vi "HDM3065B.vi"(4 "error in":T14, 7 "Command":T15) -> (0 "error out":T14, 3 "Response":T12)   [LabVIEW 2018]
uses:
  MOKO_LabViewLibrary/MokoLowLevel/MokoLowLovelControl/MLLC_Command.ctl
  MOKO_LabViewLibrary/MokoLowLevel/MokoLowLovelControl/MLLC_Error.ctl
  MOKO_LabViewLibrary/MokoLowLevel/MokoLowLovelControl/MLLC_Mode.ctl
  MOKO_LabViewLibrary/MokoLowLevel/MokoLowLovelControl/MLLC_Response.ctl
  MOKO_LabViewLibrary/MokoLowLevel/MokoLowLovelControl/MLLC_DriverName.ctl
  MOKO_LabViewLibrary/MokoLowLevel/MokoLowLovelControl/MLLC_Request.ctl
  MOKO_LabViewLibrary/MokoLowLevel/MokoLowLovelControl/MLLC_ErrorCode.ctl
  MOKO_LabViewLibrary/MokoLowLevel/MokoLowLovelControl/MLLC_ResponseInit.ctl
  MOKO_LabViewLibrary/MokoLowLevel/MokoLowLovelControl/MLLC_ConnectCluster.ctl
  MOKO_LabViewLibrary/MokoLowLevel/MokoLowLovelControl/MLLC_InterfaceType.ctl
  MOKO_LabViewLibrary/MokoLowLevel/MokoLowLovelControl/MLLC_OpenedSession.ctl
  MOKO_LabViewLibrary/MokoLowLevel/MokoLowLovelControl/MLLC_InterfaceSettings.ctl
  MOKO_LabViewLibrary/MokoLowLevel/MokoLowLovelControl/MLLC_InterfaceKind.ctl
  data/HDM3065B_Functions.ctl
panel:
  in  "Settings":T8={"Saved Data"=variant, "Data"={"Connect"={"InterfaceType"=enum."VISA", "OpenedSession"="", "InterfaceSettings"={"Interface"=enum."GPIB", "EOS 4 read"=enum."LF (\\n)", "EOS 4 write"=enum."LF (\\n)", "TMO, ms"=5000, "Sett"=variant(cluster{"Baud Rate":u32, "Data Bits":u16, "Parity":u16, "Stop Bits":u16, "Flow Control":u16, "Eho":bool} {"Baud Rate"=75, "Data Bits"=0, "Parity"=0, "Stop Bits"=0, "Flow Control"=0, "Eho"=FALSE})}}, "Channel"=1, "Func"=enum."VDC"}}
  in  "Response Init array":T9="HEWLETT-PACKARD,34401A,0,9-4-1"
  in  "Error Code":T6=5475
  in  "Request":T10="*idn?"
  in  "Driver Name":T11="HDM3065B_GERMAN"
  in  "Mode":T13=enum."Check"
  # "SCPI = MEASure:VOLTage:DC?"
  # "SCPI = SENSe:VOLTage :RANGe 20"
  # "SCPI = SENSe:VOLTage :RANGe MAX"
  # "SCPI = MEASure:VOLTage:DC?"
  # "SCPI = VOLTage :RANGe MAX"
  # "HDM3065B CUSTOM DRIVER GERMAN"
  # "MEASure | FETCh2\n:ENABle <n>\n:ARRay :CURRent?1\n:NTRansition <n>\n :VOLTage?1"
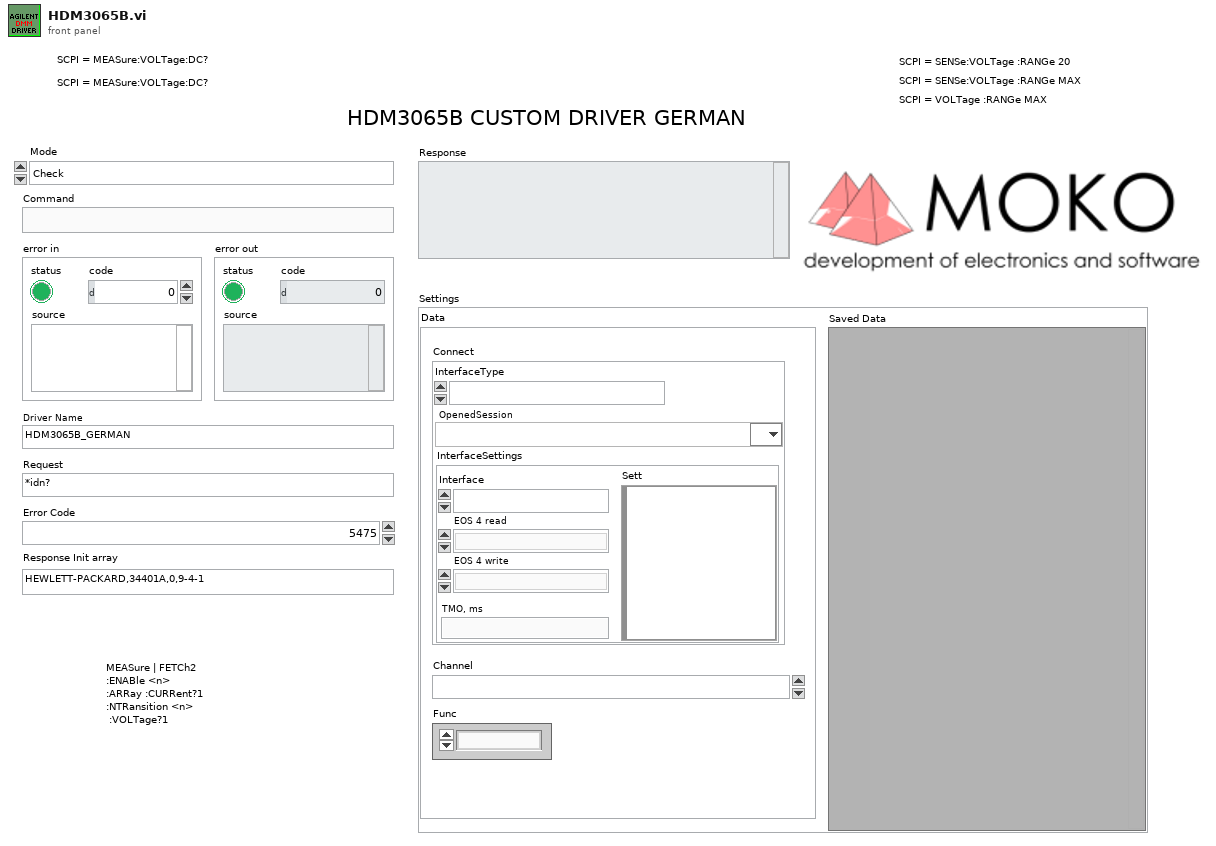
[diagram p1: front panel]
types:
  T1 = typedef "MLLC_ConnectCluster.ctl" = cluster{"InterfaceType":T2, "OpenedSession":T3, "InterfaceSettings":T4}
  T2 = typedef "MLLC_InterfaceType.ctl" = enum16{"VISA", "Prologix USB-GPIB"}
  T3 = typedef "MLLC_OpenedSession.ctl" = refnum<visa-resource-name>
  T4 = typedef "MLLC_InterfaceSettings.ctl" = cluster{"Interface":T5, "EOS 4 read":enum16{"Default (=EOS 4 write)", "CR (\\r)", "LF (\\n)", "None"}, "EOS 4 write":enum16{"CR+LF (\\r\\n)", "CR (\\r)", "LF (\\n)", "None"}, "TMO, ms":i32, "Sett":variant}
  T5 = typedef "MLLC_InterfaceKind.ctl" = enum16{"RS232", "GPIB", "USB", "Ethernet", "another"}
  T6 = typedef "MLLC_ErrorCode.ctl" = u32
  T7 = typedef "HDM3065B_Functions.ctl" = enum16{"VDC", "VAC", "IDC", "IAC", "F", "R2", "R4", "CAP"}
  T8 = cluster{"Saved Data":variant, "Data":cluster{"Connect":T1, "Channel":T6, "Func":T7}}
  T9 = typedef "MLLC_ResponseInit.ctl" = string
  T10 = typedef "MLLC_Request.ctl" = string
  T11 = typedef "MLLC_DriverName.ctl" = string
  T12 = typedef "MLLC_Response.ctl" = string
  T13 = typedef "MLLC_Mode.ctl" = enum16{"get", "set", "close", "Init", "Check"}
  T14 = typedef "MLLC_Error.ctl" = errorcluster
  T15 = typedef "MLLC_Command.ctl" = string
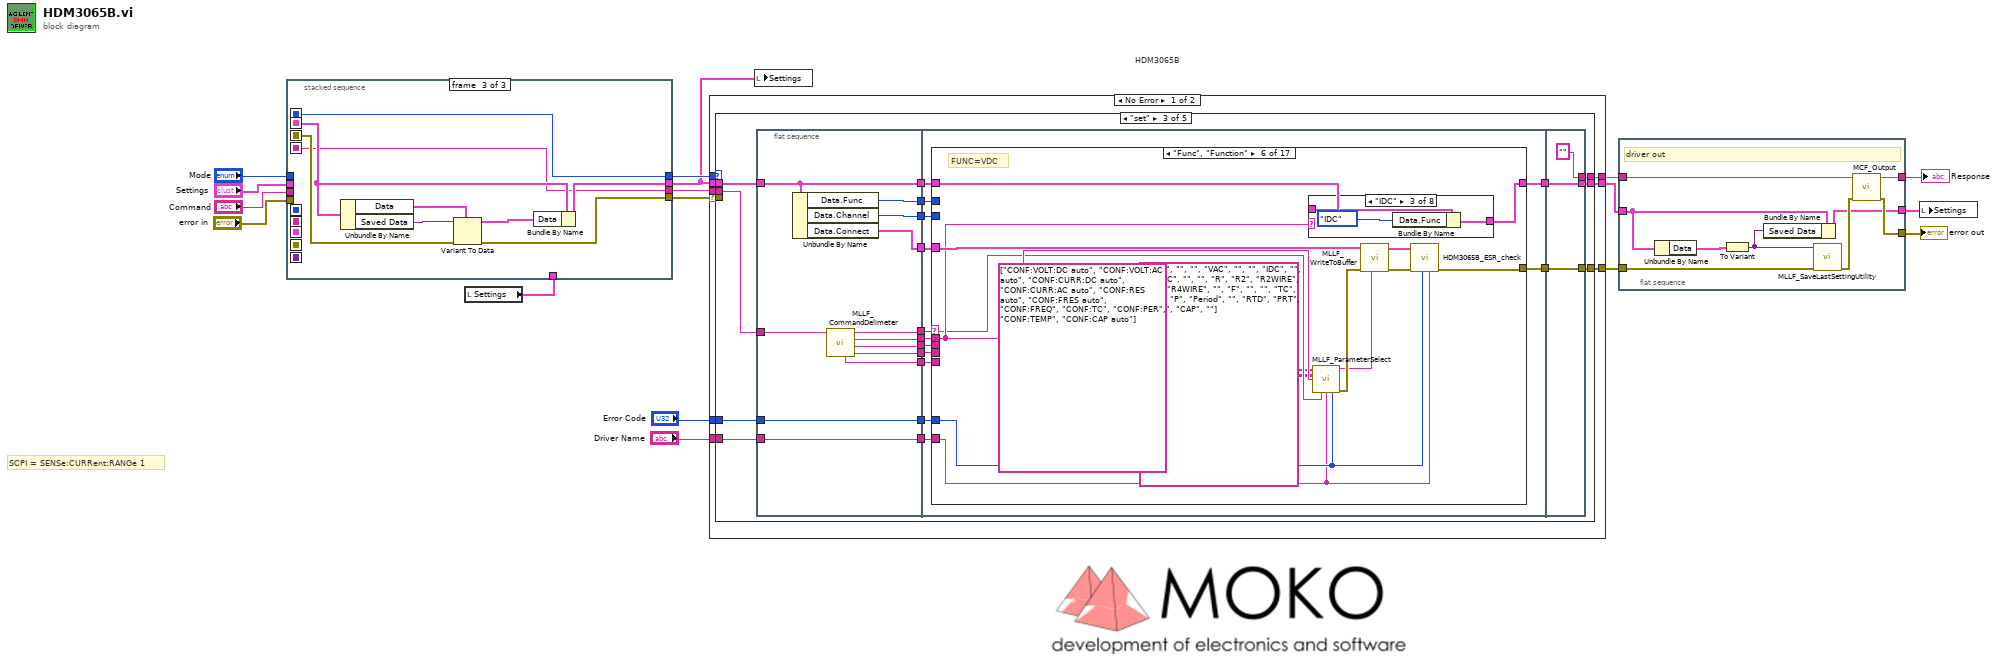
[diagram p0: block diagram]
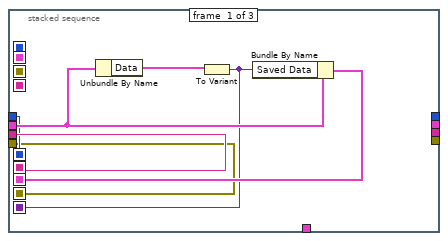
[diagram p2: hidden frame]
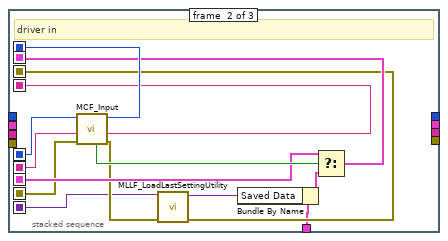
[diagram p3: hidden frame]
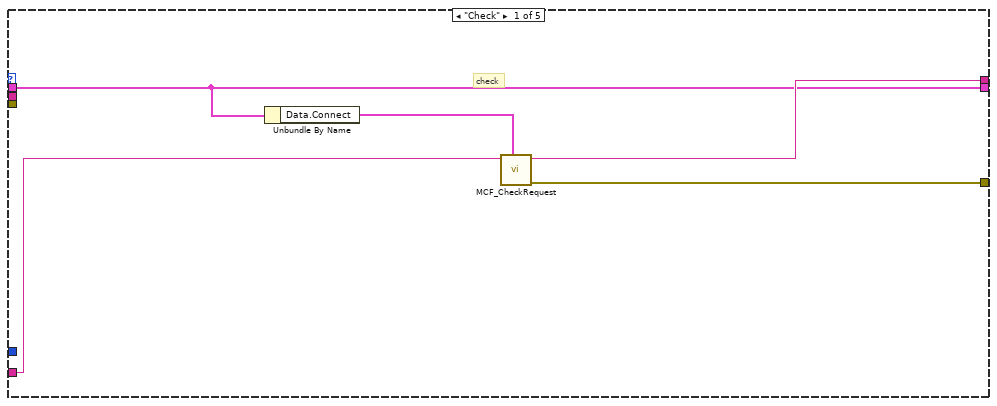
[diagram p4: hidden frame]
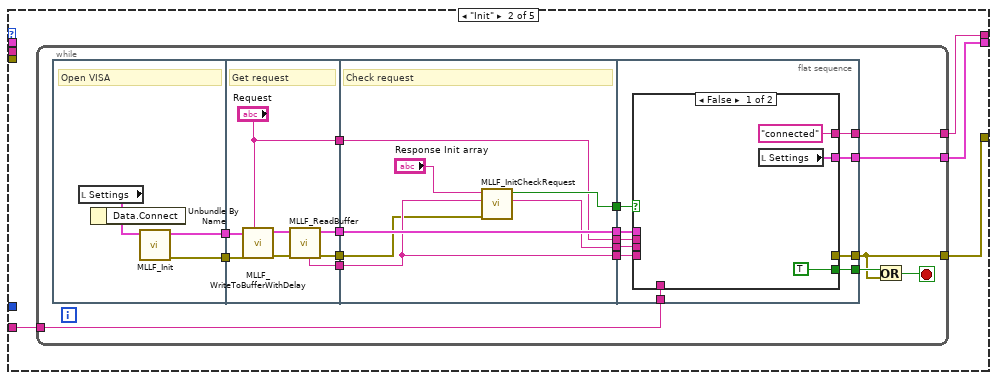
[diagram p5: hidden frame]
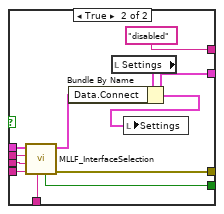
[diagram p6: hidden frame]
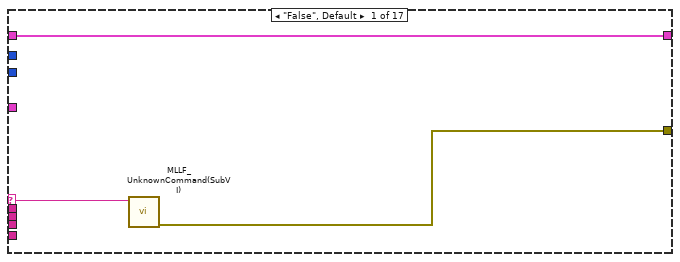
[diagram p7: hidden frame]
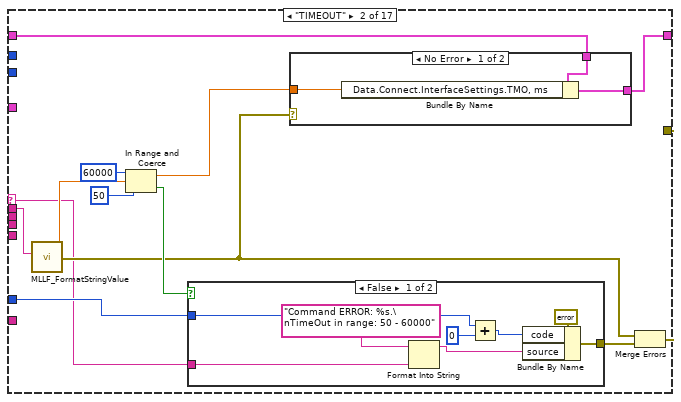
[diagram p8: hidden frame]
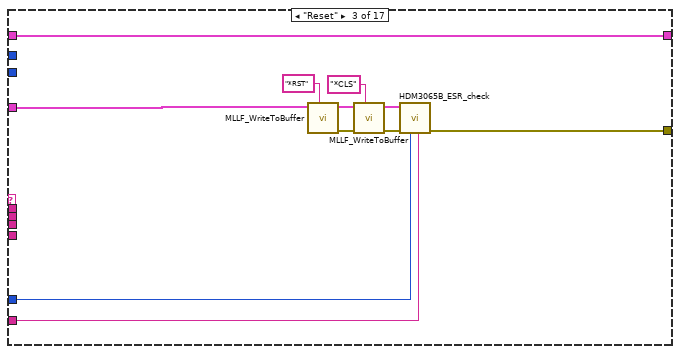
[diagram p11: hidden frame]
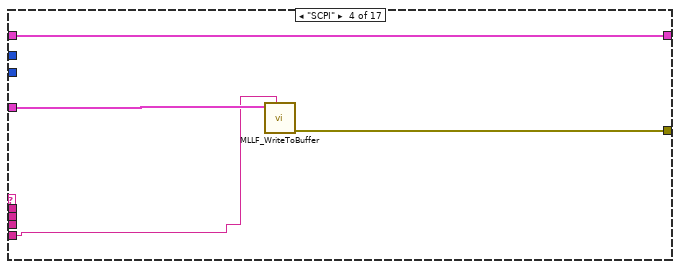
[diagram p12: hidden frame]
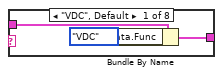
[diagram p14: hidden frame]
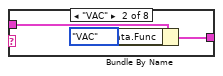
[diagram p15: hidden frame]
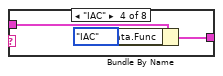
[diagram p16: hidden frame]
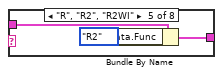
[diagram p17: hidden frame]
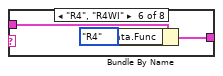
[diagram p18: hidden frame]
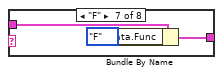
[diagram p19: hidden frame]
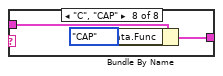
[diagram p20: hidden frame]
diagram:
  # "SCPI = SENSe:CURRent:RANGe 1"
  # "HDM3065B"
  n1 = local read "Settings"() -> (w8:T8)
  n2 = stacked-sequence {
    seq-local: [w20 _ _] -> [_ w36 _]
    seq-local: [w19 _ _] -> [_ w37 _]
    seq-local: [w22 _ _] -> [_ w32 _]
    seq-local: [w18 _ _] -> [_ w31 _]
    seq-local: [w21 _ _] -> [_ w27 _]
    seq-local: [_ w28 _] -> [_ _ w44]
    seq-local: [_ w38 _] -> [_ _ w41]
    seq-local: [_ w35 _] -> [_ _ w40]
    seq-local: [_ w34 _] -> [_ _ w45]
    tunnel: "Command" -> [w20 _ _]
    tunnel: "Mode" -> [w19 _ _]
    tunnel: "error in" -> [w18 _ _]
    tunnel: "Settings" -> [w23 _ _]
    tunnel: w8 -> [_ w26 _]
    tunnel: [_ _ w40] -> w10
    tunnel: [_ _ w43] -> w1
    tunnel: [_ _ w42] -> w9
    tunnel: [_ _ w41] -> w11
    frame #0 {
      n3 = Unbundle By Name(w23) -> ("Data"=w24:cluster{"Connect":T1, "Channel":T6, "Func":T7})
      n4 = To Variant(anything=w24) -> (Variant=w21:variant)
      n5 = Bundle By Name(cluster=w23, "Saved Data"=w21) -> (w22:T8)
    }
    frame #1 {
      # "driver in"
      n6 = call "MCF_Input.vi"("Error In"=w31, "Command in"=w36, "Mode in"=w37) -> ("Error Out"=w30:errorcluster, "Command out"=w35:string, "Mode out"=w38:T13, "Boolean"=w33:bool)  [unwired: 5 in]
      n7 = call "MLLF_LoadLastSettingUtility.vi"("Error In"=w30, "Save data in"=w27) -> ("Error Out"=w28:errorcluster, "Save data out"=w25:variant)  [unwired: 8 in]
      n8 = Bundle By Name(cluster=w26, "Saved Data"=w25) -> (w29:T8)
      n9 = Select(t=w32, s=w33, f=w29) -> (s? t:f=w34:T8)
    }
    frame #2 {
      n10 = Unbundle By Name(w45) -> ("Data"=w46:cluster{"Connect":T1, "Channel":T6, "Func":T7}, "Saved Data"=w39:variant)
      n11 = Variant To Data(error in=w44, type=w46, Variant=w39) -> (data=w47:cluster{"Connect":T1, "Channel":T6, "Func":T7}, error out=w42:errorcluster)
      n12 = Bundle By Name(cluster=w45, "Data"=w47) -> (w43:T8)
    }
  }
  n13 = case shown="No Error" w9 {
    selector: w9 -> [w53 w607]
    tunnel: [w54 w607] -> w5
    tunnel: w11 -> [w56 _]
    tunnel: [w55 "An error occurred in the driver input module." ("String")] -> w7
    tunnel: w10 -> [w48 _]
    tunnel: w1 -> [w49 w606]
    tunnel: "Error Code" -> [w52 _]
    tunnel: "Driver Name" -> [w51 _]
    tunnel: [w50 w606] -> w6
    frame No Error {
      n14 = case shown="\"set\"" w56 {
        tunnel: [w60 w65 w139 w529 "" ("String")] -> w55
        tunnel: [w61 w63 w142 w530 w603] -> w54
        tunnel: w53 -> [_ _ _ w544 _]
        tunnel: w52 -> [_ _ w145 w546 _]
        tunnel: w51 -> [w59 w62 w143 w545 _]
        tunnel: [w57 w64 w144 w547 w602] -> w50
        tunnel: w49 -> [w57 _ w128 w535 w602]
        tunnel: w48 -> [_ _ w127 w534 _]
        frame "Check" {
          # "check"
          n15 = Unbundle By Name(w57) -> ("Data.Connect"=w58:T1)
          n16 = call "MCF_CheckRequest.vi"("Permanent data.Connect"=w58, "Driver Name"=w59) -> ("Error Out"=w61:errorcluster, "Output String"=w60:string)  [unwired: 8 in]
        }
        frame "Init" {
          n17 = while {
            tunnel: [w71] -> w63
            tunnel: [w70] -> w65
            tunnel: [w69] -> w64
            tunnel: w62 -> [w73]
            stop <- w82 stop-if-true
            n18 = flat-sequence {
              tunnel: [w86] -> w81
              tunnel: [w85] -> w80
              tunnel: w81 -> [w92]
              tunnel: w80 -> [w91]
              tunnel: [w90] -> w79
              tunnel: [w89] -> w78
              tunnel: [w88] -> w77
              tunnel: ["Request"] -> w67
              tunnel: w79 -> [w98]
              tunnel: w78 -> [w101]
              tunnel: w77 -> [w100]
              tunnel: [w101] -> w76
              tunnel: [w100] -> w75
              tunnel: [w97] -> w74
              tunnel: [w96] -> w68
              tunnel: w67 -> [w95]
              tunnel: [w95] -> w66
              tunnel: w76 -> [w110]
              tunnel: w75 -> [w109]
              tunnel: w74 -> [w111]
              tunnel: w73 -> [w108]
              tunnel: [w107] -> w72
              tunnel: [w106] -> w71
              tunnel: [w105] -> w70
              tunnel: [w104] -> w69
              tunnel: w68 -> [w103]
              tunnel: w66 -> [w102]
              frame #0 {
                # "Open VISA"
                n19 = local read "Settings"() -> (w84:T8)
                n20 = Unbundle By Name(w84) -> ("Data.Connect"=w83:T1)
                n21 = call "MLLF_Init.vi"("DriverConnect in"=w83) -> ("Error Out"=w86:errorcluster, "DriverConnect out"=w85:T1)  [unwired: 7 in]
              }
              frame #1 {
                # "Get request"
                n22 = call "MLLF_WriteToBufferWithDelay.vi"("Command"="Request", "Error In"=w92, "DriverConnect in"=w91) -> ("Error Out"=w93:errorcluster, "DriverConnect out"=w94:T1)  [unwired: 7 in]
                n23 = call "MLLF_ReadBuffer.vi"("Error In"=w93, "DriverConnect in"=w94) -> ("Error Out"=w90:errorcluster, "DriverConnect out"=w89:T1, "String"=w88:string)  [unwired: 6 in]
              }
              frame #2 {
                # "Check request"
                n24 = call "MLLF_InitCheckRequest.vi"("error in (no error)"=w98, "Answer"=w100, "Response Init"="Response Init array") -> ("ResponseInit out"=w96:string, "Design"=w97:bool)  [unwired: 5 in, 2 out]
              }
              frame #3 {
                n25 = case shown="False" w111 {
                  tunnel: w110 -> [_ w124]
                  tunnel: [TRUE w119] -> w107
                  tunnel: [_ w122] -> w106
                  tunnel: ["connected" "disabled"] -> w105
                  tunnel: [w112 w120] -> w104
                  tunnel: w109 -> [_ w117]
                  tunnel: w108 -> [_ w118]
                  tunnel: w103 -> [_ w116]
                  tunnel: w102 -> [_ w115]
                  frame False {
                    n26 = local read "Settings"() -> (w112:T8)
                  }
                  frame True {
                    n27 = call "MLLF_InterfaceSelection.vi"("Driver Name"=w118, "Answer:"=w117, "Response"=w116, "Request"=w115, "DriverConnect in"=w124) -> ("error out"=w122:T14, "DriverConnect out"=w123:T1, "stop init?"=w119:bool)  [unwired: 2 in, 2 out]
                    n28 = local read "Settings"() -> (w125:T8)
                    n29 = Bundle By Name(cluster=w125, "Data.Connect"=w123) -> (w120:T8)
                    n30 = local write "Settings"(w120) -> ()
                  }
                }
              }
            }
            n31 = Or(x=w72, y=w71) -> (x .or. y?=w82:bool)
          }
        }
        frame "set" {
          n32 = flat-sequence {
            tunnel: w143 -> [w156]
            tunnel: w128 -> [w147]
            tunnel: w145 -> [w157]
            tunnel: [w157] -> w138
            tunnel: [w147] -> w137
            tunnel: [w156] -> w136
            tunnel: [w153] -> w135
            tunnel: [w154] -> w134
            tunnel: [w155] -> w133
            tunnel: [w148] -> w132
            tunnel: [w149] -> w131
            tunnel: [w150] -> w130
            tunnel: [w151] -> w129
            tunnel: w127 -> [w152]
            tunnel: [w146] -> w126
            tunnel: [w168] -> w141
            tunnel: [w161] -> w140
            tunnel: w138 -> [w170]
            tunnel: w137 -> [w169]
            tunnel: w136 -> [w167]
            tunnel: w135 -> [w166]
            tunnel: w134 -> [w165]
            tunnel: w133 -> [w164]
            tunnel: w132 -> [w163]
            tunnel: w131 -> [w162]
            tunnel: w130 -> [w160]
            tunnel: w129 -> [w159]
            tunnel: w126 -> [w158]
            tunnel: [w527] -> w142
            tunnel: [w528] -> w144
            tunnel: w141 -> [w528]
            tunnel: w140 -> [w527]
            tunnel: ["" ("String")] -> w139
            frame #0 {
              n33 = Unbundle By Name(w147) -> ("Data.Func"=w155:T7, "Data.Channel"=w154:T6, "Data.Connect"=w153:T1)
              n34 = call "MLLF_CommandDelimeter.vi"("command with param"=w152) -> ("param 3"=w151:string, "param 2"=w150:string, "param 1"=w149:string, "command"=w148:string, "Spit delimetre"=w146:string)  [unwired: 6 in]
            }
            frame #1 {
              n35 = case shown="\"Func\", \"Function\"" w163 {
                selector: w163 -> [w172 w175 _ _ _ w221 _ _ _ _ _ _ w441 w448 w474 w500 w513]
                tunnel: w162 -> [_ w174 _ _ _ w222 w270 _ w303 w318 w365 w399 w442 w449 w475 w501 w514]
                tunnel: [w171 w180 w200 w210 _ w226 w253 _ w307 w336 w369 w403 w446 w470 w496 w509 w520] -> w161
                tunnel: w170 -> [_ w181 w202 _ _ w228 _ _ w306 w335 w368 w402 w443 w453 w479 w505 w522]
                tunnel: w169 -> [w173 w185 w209 w213 w214 w224 w272 w284 w308 w337 w370 w404 w447 w471 w497 w510 w525]
                tunnel: [w173 w186 w209 w213 w214 w223 w272 w284 w308 w337 w370 w404 w447 w471 w497 w510 w525] -> w168
                tunnel: w166 -> [_ _ w199 w212 _ w225 w271 _ w304 w333 w366 w400 w445 w469 w495 w503 w518]
                tunnel: w167 -> [_ _ w201 _ _ w227 _ _ w305 w334 w367 w401 w444 w454 w480 w506 w521]
                tunnel: w165 -> [_ _ _ _ _ _ _ _ _ _ _ _ _ _ _ _ _]
                tunnel: w164 -> [_ _ _ _ _ _ _ _ _ _ _ _ _ _ _ _ _]
                tunnel: w160 -> [_ _ _ _ _ _ _ _ _ _ _ _ _ _ _ _ _]
                tunnel: w159 -> [_ _ _ _ _ _ _ _ _ _ _ _ _ _ _ _ _]
                tunnel: w158 -> [_ _ _ w211 _ _ _ _ _ _ _ _ _ _ _ _ _]
                frame "False", Default {
                  n36 = call "MLLF_UnknownCommand(SubVI).vi"("Unknown command"=w172) -> ("error out"=w171:errorcluster)  [unwired: 10 in]
                }
                frame "TIMEOUT" {
                  n37 = call "MLLF_FormatStringValue.vi"("String Value"=w174) -> ("error out"=w176:T14, "number"=w177:dbl)  [unwired: 8 in, 1 out]
                  n38 = In Range and Coerce(upper limit=60000, x=w177, lower limit=50) -> (coerced(x)=w182:dbl, In Range?=w178:bool)
                  n39 = case shown="False" w178 {
                    tunnel: [w193 _] -> w179
                    tunnel: w181 -> [w192 _]
                    tunnel: w175 -> [w191 _]
                    frame False {
                      n40 = Format Into String(format string="Command ERROR: %s.\nTimeOut in range: 50 - 60000", w191) -> (resulting string=w195:string)  [unwired: 2 in, 1 out]
                      n41 = Add(x=w192, y=0) -> (x+y=w196:T6)
                      n42 = Bundle By Name(cluster=errorcluster {"status"=TRUE, "code"=0, "source"=""} ("error out"), "code"=w196, "source"=w195) -> (w193:errorcluster)
                    }
                    frame True {
                    }
                  }
                  n43 = case shown="No Error" w176 {
                    tunnel: [w189 w190] -> w186
                    tunnel: w185 -> [w188 w190]
                    tunnel: w182 -> [w187 _]
                    frame No Error {
                      n44 = Bundle By Name(cluster=w188, "Data.Connect.InterfaceSettings.TMO, ms"=w187) -> (w189:T8)
                    }
                    frame Error {
                    }
                  }
                  n45 = Merge Errors(w176, w179) -> (w180:errorcluster)
                }
                frame "Reset" {
                  n46 = call "MLLF_WriteToBuffer.vi"("String"="*RST", "DriverConnect in"=w199) -> ("error out"=w207:T14, "DriverConnect out"=w208:T1)  [unwired: 6 in]
                  n47 = call "MLLF_WriteToBuffer.vi"("String"="*CLS" ("write buffer"), "error in"=w207, "DriverConnect in"=w208) -> ("error out"=w204:T14, "DriverConnect out"=w203:T1)  [unwired: 5 in]
                  n48 = call "HDM3065B_ESR_check.vi"("Driver Name"=w201, "Error Code"=w202, "error in"=w204, "DriverConnect in"=w203) -> ("error out"=w200:T14)  [unwired: 6 in, 1 out]
                }
                frame "SCPI" {
                  n49 = call "MLLF_WriteToBuffer.vi"("String"=w211, "DriverConnect in"=w212) -> ("error out"=w210:T14)  [unwired: 6 in, 1 out]
                }
                frame "<----MAIN FUNCTIONS---->" {
                }
                frame "Func", "Function" {
                  # "FUNC=VDC"
                  n50 = case shown="\"IDC\"" w222 {
                    tunnel: w224 -> [w231 w234 w237 w240 w243 w246 w249 w252]
                    tunnel: [w230 w233 w236 w239 w242 w245 w248 w251] -> w223
                    frame "VDC", Default {
                      n51 = Bundle By Name(cluster=w231, "Data.Func"=HDM3065B_Functions."VDC" ("Func")) -> (w230:T8)
                    }
                    frame "VAC" {
                      n52 = Bundle By Name(cluster=w234, "Data.Func"=HDM3065B_Functions."VAC" ("Func")) -> (w233:T8)
                    }
                    frame "IDC" {
                      n53 = Bundle By Name(cluster=w237, "Data.Func"=HDM3065B_Functions."IDC" ("Func")) -> (w236:T8)
                    }
                    frame "IAC" {
                      n54 = Bundle By Name(cluster=w240, "Data.Func"=HDM3065B_Functions."IAC" ("Func")) -> (w239:T8)
                    }
                    frame "R", "R2", "R2WI" {
                      n55 = Bundle By Name(cluster=w243, "Data.Func"=HDM3065B_Functions."R2" ("Func")) -> (w242:T8)
                    }
                    frame "R4", "R4WI" {
                      n56 = Bundle By Name(cluster=w246, "Data.Func"=HDM3065B_Functions."R4" ("Func")) -> (w245:T8)
                    }
                    frame "F" {
                      n57 = Bundle By Name(cluster=w249, "Data.Func"=HDM3065B_Functions."F" ("Func")) -> (w248:T8)
                    }
                    frame "C", "CAP" {
                      n58 = Bundle By Name(cluster=w252, "Data.Func"=HDM3065B_Functions."CAP" ("Func")) -> (w251:T8)
                    }
                  }
                  n59 = call "MLLF_ParameterSelect.vi"("Command to equipment"=string[] ["CONF:VOLT:DC auto", "CONF:VOLT:AC auto", "CONF:CURR:DC auto", "CONF:CURR:AC auto", "CONF:RES auto", "CONF:FRES auto", "CONF:FREQ", "CONF:TC", "CONF:PER", "CONF:TEMP", "CONF:CAP auto"] ("Names"), "Names"=string[][] [["VDC", "", ""], ["VAC", "", ""], ["IDC", "", ""], ["IAC", "", ""], ["R", "R2", "R2WIRE"], ["R4", "R4WIRE", ""], ["F", "", ""], ["TC", "", ""], ["P", "Period", ""], ["RTD", "PRT", ""], ["C", "CAP", ""]], "Input"=w222, "Command"=w221, "Driver Name"=w227, "Error Code"=w228) -> ("Choice"=w215:string, "Error Out"=w216:errorcluster)  [unwired: 8 in]
                  n60 = call "MLLF_WriteToBuffer.vi"("String"=w215, "error in"=w216, "DriverConnect in"=w225) -> ("error out"=w220:T14, "DriverConnect out"=w219:T1)  [unwired: 5 in]
                  n61 = call "HDM3065B_ESR_check.vi"("Driver Name"=w227, "Error Code"=w228, "error in"=w220, "DriverConnect in"=w219) -> ("error out"=w226:T14)  [unwired: 6 in, 1 out]
                }
                frame "Range" {
                  w258 = TRUE ("replace all? (F)")
                  n62 = call "MLLF_WriteToBuffer.vi"("String"="CONFigure? ", "DriverConnect in"=w271) -> ("error out"=w266:T14, "DriverConnect out"=w267:T1)  [unwired: 6 in]
                  n63 = call "MLLF_ReadBuffer.vi"("Error In"=w266, "DriverConnect in"=w267) -> ("Error Out"=w255:errorcluster, "DriverConnect out"=w265:T1, "String"=w260:string)  [unwired: 6 in]
                  n64 = case shown="\"False\", Default" w270 {
                    selector: w270 -> [w274 _ _ _]
                    tunnel: [w277 w278 w280 w282] -> w269
                    tunnel: [w276 "RANG:AUTO ON" ("String") "RANG MIN" ("String") "RANG MAX" ("String")] -> w263
                    tunnel: w255 -> [w273 w278 w280 w282]
                    frame "False", Default {
                      n65 = call "MLLF_FormatStringValue.vi"("error in"=w273, "String Value"=w274, "Format"="RANG %#e" ("format string")) -> ("error out"=w277:T14, "String Value Formated"=w276:T15)  [unwired: 6 in, 1 out]
                    }
                    frame "Auto" {
                    }
                    frame "MIN" {
                    }
                    frame "MAX" {
                    }
                  }
                  n66 = Search and Replace String(replace all?=w258, case sensitive?=w258, input string=w260, search string="\"") -> (result string=w259:string)  [unwired: 4 in, 3 out]
                  n67 = Match Pattern(string=w259, regular expression="[\\s\\t]+") -> (before substring=w261:string)  [unwired: 1 in, 3 out]
                  n68 = Concatenate Strings("SENSe:" ("string"), w261, ":" ("string"), w263) -> (w256:string)
                  n69 = call "MLLF_WriteToBuffer.vi"("String"=w256, "error in"=w269, "DriverConnect in"=w265) -> ("error out"=w253:T14)  [unwired: 5 in, 1 out]
                }
                frame "---------ADDITIONAL---------" {
                }
                frame "Res", "Resolution" {
                  w288 = TRUE ("replace all? (F)")
                  n70 = call "MLLF_WriteToBuffer.vi"("String"="CONFigure? ", "DriverConnect in"=w304) -> ("error out"=w297:T14, "DriverConnect out"=w298:T1)  [unwired: 6 in]
                  n71 = call "MLLF_ReadBuffer.vi"("Error In"=w297, "DriverConnect in"=w298) -> ("Error Out"=w296:errorcluster, "DriverConnect out"=w295:T1, "String"=w290:string)  [unwired: 6 in]
                  n72 = Search and Replace String(replace all?=w288, case sensitive?=w288, input string=w290, search string="\"") -> (result string=w289:string)  [unwired: 4 in, 3 out]
                  n73 = case shown="\"MIN\"" w303 {
                    selector: w303 -> [w310 _ _]
                    tunnel: [w313 w314 w316] -> w302
                    tunnel: [w312 "RES MAX" ("String") "RES MIN" ("String")] -> w293
                    tunnel: w296 -> [w309 w314 w316]
                    frame "False", Default {
                      n74 = call "MLLF_FormatStringValue.vi"("error in"=w309, "String Value"=w310, "Format"="RES %#e" ("format string")) -> ("error out"=w313:T14, "String Value Formated"=w312:T15)  [unwired: 6 in, 1 out]
                    }
                    frame "MAX" {
                    }
                    frame "MIN" {
                    }
                  }
                  n75 = Match Pattern(string=w289, regular expression="[\\s\\t]+") -> (before substring=w291:string)  [unwired: 1 in, 3 out]
                  n76 = Concatenate Strings("SENSe:" ("string"), w291, ":" ("string"), w293) -> (w286:string)
                  n77 = call "MLLF_WriteToBuffer.vi"("String"=w286, "error in"=w302, "DriverConnect in"=w295) -> ("error out"=w301:T14, "DriverConnect out"=w300:T1)  [unwired: 5 in]
                  n78 = call "HDM3065B_ESR_check.vi"("Driver Name"=w305, "Error Code"=w306, "error in"=w301, "DriverConnect in"=w300) -> ("error out"=w307:T14)  [unwired: 6 in, 1 out]
                }
                frame "Aper", "Aperture", "MeasTime" {
                  w321 = TRUE ("replace all? (F)")
                  n79 = call "MLLF_WriteToBuffer.vi"("String"="CONFigure? ", "DriverConnect in"=w333) -> ("error out"=w330:T14, "DriverConnect out"=w331:T1)  [unwired: 6 in]
                  n80 = call "MLLF_ReadBuffer.vi"("Error In"=w330, "DriverConnect in"=w331) -> ("Error Out"=w329:errorcluster, "DriverConnect out"=w328:T1, "String"=w323:string)  [unwired: 6 in]
                  n81 = Search and Replace String(replace all?=w321, case sensitive?=w321, input string=w323, search string="\"") -> (result string=w322:string)  [unwired: 4 in, 3 out]
                  n82 = case shown="\"OFF\"" w318 {
                    selector: w318 -> [w342 _]
                    tunnel: [w345 w346] -> w340
                    tunnel: [w344 "APER:ENAB OFF" ("String")] -> w326
                    tunnel: w329 -> [w341 w346]
                    frame "False", Default {
                      n83 = call "MLLF_FormatStringValue.vi"("error in"=w341, "String Value"=w342, "Format"="APER %#e" ("format string")) -> ("error out"=w345:T14, "String Value Formated"=w344:T15)  [unwired: 6 in, 1 out]
                    }
                    frame "OFF" {
                    }
                  }
                  n84 = Match Pattern(string=w322, regular expression="[\\s\\t]+") -> (before substring=w324:string)  [unwired: 1 in, 3 out]
                  n85 = Concatenate Strings(w324, ":" ("string"), w326) -> (w319:string)
                  n86 = call "MLLF_WriteToBuffer.vi"("String"=w319, "error in"=w340, "DriverConnect in"=w328) -> ("error out"=w339:T14, "DriverConnect out"=w338:T1)  [unwired: 5 in]
                  n87 = call "HDM3065B_ESR_check.vi"("Driver Name"=w334, "Error Code"=w335, "error in"=w339, "DriverConnect in"=w338) -> ("error out"=w336:T14)  [unwired: 6 in, 1 out]
                }
                frame "IntegrationTime", "IntTime", "NPLC" {
                  w351 = TRUE ("replace all? (F)")
                  n88 = call "MLLF_WriteToBuffer.vi"("String"="CONFigure? ", "DriverConnect in"=w366) -> ("error out"=w359:T14, "DriverConnect out"=w360:T1)  [unwired: 6 in]
                  n89 = call "MLLF_ReadBuffer.vi"("Error In"=w359, "DriverConnect in"=w360) -> ("DriverConnect out"=w358:T1, "String"=w353:string)  [unwired: 6 in, 1 out]
                  n90 = Search and Replace String(replace all?=w351, case sensitive?=w351, input string=w353, search string="\"") -> (result string=w352:string)  [unwired: 4 in, 3 out]
                  n91 = case shown="Default" w365 {
                    tunnel: [w374 w378 w382] -> w364
                    tunnel: [w373 w377 w381] -> w356
                    tunnel: w365 -> [w371 w375 w379]
                    frame Default {
                      n92 = call "MLLF_FormatStringValue.vi"("String Value"=w371, "Format"="NPLC %#e" ("format string")) -> ("error out"=w374:T14, "String Value Formated"=w373:T15)  [unwired: 7 in, 1 out]
                    }
                    frame "MIN" {
                      n93 = call "MLLF_FormatStringValue.vi"("String Value"=w375, "Format"="NPLC MIN" ("format string")) -> ("error out"=w378:T14, "String Value Formated"=w377:T15)  [unwired: 7 in, 1 out]
                    }
                    frame "MAX" {
                      n94 = call "MLLF_FormatStringValue.vi"("String Value"=w379, "Format"="NPLC MAX" ("format string")) -> ("error out"=w382:T14, "String Value Formated"=w381:T15)  [unwired: 7 in, 1 out]
                    }
                  }
                  n95 = Match Pattern(string=w352, regular expression="[\\s\\t]+") -> (before substring=w354:string)  [unwired: 1 in, 3 out]
                  n96 = Concatenate Strings("SENSe:" ("string"), w354, ":" ("string"), w356) -> (w349:string)
                  n97 = call "MLLF_WriteToBuffer.vi"("String"=w349, "error in"=w364, "DriverConnect in"=w358) -> ("error out"=w363:T14, "DriverConnect out"=w362:T1)  [unwired: 5 in]
                  n98 = call "HDM3065B_ESR_check.vi"("Driver Name"=w367, "Error Code"=w368, "error in"=w363, "DriverConnect in"=w362) -> ("error out"=w369:T14)  [unwired: 6 in, 1 out]
                }
                frame "ACBand", "ACBandwidth", "Band", "Bandwidth" {
                  w386 = TRUE ("replace all? (F)")
                  n99 = call "MLLF_WriteToBuffer.vi"("String"="CONFigure? ", "DriverConnect in"=w400) -> ("error out"=w393:T14, "DriverConnect out"=w394:T1)  [unwired: 6 in]
                  n100 = call "MLLF_ReadBuffer.vi"("Error In"=w393, "DriverConnect in"=w394) -> ("Error Out"=w392:errorcluster, "DriverConnect out"=w391:T1, "String"=w388:string)  [unwired: 6 in]
                  n101 = case shown="\"MAX\"" w399 {
                    tunnel: [w409 w414 w419] -> w398
                    tunnel: w392 -> [w408 w413 w418]
                    tunnel: [w407 w412 w417] -> w389
                    tunnel: w399 -> [w405 w410 w415]
                    frame Default {
                      n102 = call "MLLF_FormatStringValue.vi"("error in"=w408, "String Value"=w405, "Format"="BAND %#f" ("format string")) -> ("error out"=w409:T14, "String Value Formated"=w407:T15)  [unwired: 6 in, 1 out]
                    }
                    frame "MAX" {
                      n103 = call "MLLF_FormatStringValue.vi"("error in"=w413, "String Value"=w410, "Format"="BAND MAX" ("format string")) -> ("error out"=w414:T14, "String Value Formated"=w412:T15)  [unwired: 6 in, 1 out]
                    }
                    frame "MIN" {
                      n104 = call "MLLF_FormatStringValue.vi"("error in"=w418, "String Value"=w415, "Format"="BAND MIN" ("format string")) -> ("error out"=w419:T14, "String Value Formated"=w417:T15)  [unwired: 6 in, 1 out]
                    }
                  }
                  n105 = Search and Replace String(replace all?=w386, case sensitive?=w386, input string=w388, search string="\"") -> (result string=w387:string)  [unwired: 4 in, 3 out]
                  n106 = Match Pattern(string=w387, regular expression="[\\s\\t]+") -> ()  [unwired: 1 in, 4 out]
                  n107 = Concatenate Strings(":DET:" ("string"), w389) -> (w384:string)
                  n108 = call "MLLF_WriteToBuffer.vi"("String"=w384, "error in"=w398, "DriverConnect in"=w391) -> ("error out"=w397:T14, "DriverConnect out"=w396:T1)  [unwired: 5 in]
                  n109 = call "HDM3065B_ESR_check.vi"("Driver Name"=w401, "Error Code"=w402, "error in"=w397, "DriverConnect in"=w396) -> ("error out"=w403:T14)  [unwired: 6 in, 1 out]
                }
                frame "AutoZero", "ZERO" {
                  w429 = TRUE ("replace all? (F)")
                  n110 = call "MLLF_WriteToBuffer.vi"("String"="CONFigure? ", "DriverConnect in"=w445) -> ("error out"=w436:T14, "DriverConnect out"=w437:T1)  [unwired: 6 in]
                  n111 = call "MLLF_ReadBuffer.vi"("Error In"=w436, "DriverConnect in"=w437) -> ("Error Out"=w423:errorcluster, "DriverConnect out"=w435:T1, "String"=w431:string)  [unwired: 6 in]
                  n112 = Search and Replace String(replace all?=w429, case sensitive?=w429, input string=w431, search string="\"") -> (result string=w430:string)  [unwired: 4 in, 3 out]
                  n113 = Match Pattern(string=w430, regular expression="[\\s\\t]+") -> (before substring=w432:string)  [unwired: 1 in, 3 out]
                  n114 = call "MLLF_ParameterSelect.vi"("Command to equipment"=string[] ["ZERO:AUTO OFF", "ZERO:AUTO ON", "ZERO:AUTO ONCE"] ("Names"), "Ignor case(default = true)"=TRUE, "Names"=string[][] [["OFF"], ["ON"], ["ONCE"]], "Input"=w442, "Error In"=w423, "Command"=w441, "Driver Name"=w444, "Error Code"=w443) -> ("Choice"=w422:string, "Error Out"=w424:errorcluster)  [unwired: 6 in]
                  n115 = Concatenate Strings("SENSe:" ("string"), w432, ":" ("string"), w422) -> (w427:string)
                  n116 = call "MLLF_WriteToBuffer.vi"("String"=w427, "error in"=w424, "DriverConnect in"=w435) -> ("error out"=w440:T14, "DriverConnect out"=w439:T1)  [unwired: 5 in]
                  n117 = call "HDM3065B_ESR_check.vi"("Driver Name"=w444, "Error Code"=w443, "error in"=w440, "DriverConnect in"=w439) -> ("error out"=w446:T14)  [unwired: 6 in, 1 out]
                }
                frame "LOWPOWER" {
                  w459 = TRUE ("replace all? (F)")
                  n118 = call "MLLF_WriteToBuffer.vi"("String"="CONFigure? ", "DriverConnect in"=w469) -> ("error out"=w466:T14, "DriverConnect out"=w467:T1)  [unwired: 6 in]
                  n119 = call "MLLF_ReadBuffer.vi"("Error In"=w466, "DriverConnect in"=w467) -> ("Error Out"=w451:errorcluster, "DriverConnect out"=w465:T1, "String"=w461:string)  [unwired: 6 in]
                  n120 = Search and Replace String(replace all?=w459, case sensitive?=w459, input string=w461, search string="\"") -> (result string=w460:string)  [unwired: 4 in, 3 out]
                  n121 = Match Pattern(string=w460, regular expression="[\\s\\t]+") -> (before substring=w462:string)  [unwired: 1 in, 3 out]
                  n122 = call "MLLF_ParameterSelect.vi"("Command to equipment"=string[] ["POW:LIM OFF", "POW:LIM ON"] ("Names"), "Names"=string[][] [["0", "DIS", "DISABLE", "DISABLED", "OFF"], ["1", "EN", "ENABLE", "ENABLED", "ON"]], "Input"=w449, "Error In"=w451, "Command"=w448, "Driver Name"=w454, "Error Code"=w453) -> ("Choice"=w450:string, "Error Out"=w452:errorcluster)  [unwired: 7 in]
                  n123 = Concatenate Strings(w462, ":" ("string"), w450) -> (w457:string)
                  n124 = call "MLLF_WriteToBuffer.vi"("String"=w457, "error in"=w452, "DriverConnect in"=w465) -> ("error out"=w473:T14, "DriverConnect out"=w472:T1)  [unwired: 5 in]
                  n125 = call "HDM3065B_ESR_check.vi"("Driver Name"=w454, "Error Code"=w453, "error in"=w473, "DriverConnect in"=w472) -> ("error out"=w470:T14)  [unwired: 6 in, 1 out]
                }
                frame "VOLTAGELIMITED" {
                  w485 = TRUE ("replace all? (F)")
                  n126 = call "MLLF_WriteToBuffer.vi"("String"="CONFigure? ", "DriverConnect in"=w495) -> ("error out"=w492:T14, "DriverConnect out"=w493:T1)  [unwired: 6 in]
                  n127 = call "MLLF_ReadBuffer.vi"("Error In"=w492, "DriverConnect in"=w493) -> ("Error Out"=w477:errorcluster, "DriverConnect out"=w491:T1, "String"=w487:string)  [unwired: 6 in]
                  n128 = Search and Replace String(replace all?=w485, case sensitive?=w485, input string=w487, search string="\"") -> (result string=w486:string)  [unwired: 4 in, 3 out]
                  n129 = Match Pattern(string=w486, regular expression="[\\s\\t]+") -> (before substring=w488:string)  [unwired: 1 in, 3 out]
                  n130 = call "MLLF_ParameterSelect.vi"("Command to equipment"=string[] ["VOLT:LIM OFF", "VOLT:LIM ON"] ("Names"), "Names"=string[][] [["0", "DIS", "DISABLE", "DISABLED", "OFF"], ["1", "EN", "ENABLE", "ENABLED", "ON"]], "Input"=w475, "Error In"=w477, "Command"=w474, "Driver Name"=w480, "Error Code"=w479) -> ("Choice"=w476:string, "Error Out"=w478:errorcluster)  [unwired: 7 in]
                  n131 = Concatenate Strings(w488, ":" ("string"), w476) -> (w483:string)
                  n132 = call "MLLF_WriteToBuffer.vi"("String"=w483, "error in"=w478, "DriverConnect in"=w491) -> ("error out"=w499:T14, "DriverConnect out"=w498:T1)  [unwired: 5 in]
                  n133 = call "HDM3065B_ESR_check.vi"("Driver Name"=w480, "Error Code"=w479, "error in"=w499, "DriverConnect in"=w498) -> ("error out"=w496:T14)  [unwired: 6 in, 1 out]
                }
                frame "FILT", "FILTER" {
                  # "FILT=DIS"
                  n134 = call "MLLF_ParameterSelect.vi"("Command to equipment"=string[] ["INPut:FILTer:STATE OFF", "INPut:FILTer:STATE ON"] ("Names"), "Names"=string[][] [["0", "DIS", "DISABLE", "DISABLED", "OFF"], ["1", "EN", "ENABLE", "ENABLED", "ON"]], "Input"=w501, "Command"=w500, "Driver Name"=w506, "Error Code"=w505) -> ("Choice"=w502:string, "Error Out"=w504:errorcluster)  [unwired: 8 in]
                  n135 = call "MLLF_WriteToBuffer.vi"("String"=w502, "error in"=w504, "DriverConnect in"=w503) -> ("error out"=w512:T14, "DriverConnect out"=w511:T1)  [unwired: 5 in]
                  n136 = call "HDM3065B_ESR_check.vi"("Driver Name"=w506, "Error Code"=w505, "error in"=w512, "DriverConnect in"=w511) -> ("error out"=w509:T14)  [unwired: 6 in, 1 out]
                }
                frame "SND", "Sound" {
                  # "sound"
                  # "sound=off"
                  n137 = call "MLLF_ParameterSelect.vi"("Command to equipment"=string[] ["SYST:BEEP:STAT OFF", "SYST:BEEP:STAT ON", "SYST:BEEP"] ("Names"), "Names"=string[][] [["0", "DIS", "DISABLED", "DISABLE", "OFF"], ["1", "EN", "ENABLE", "ENABLED", "ON"], [" ", "", "", "", ""]], "Input"=w514, "Command"=w513, "Driver Name"=w521, "Error Code"=w522) -> ("Choice"=w517:string, "Error Out"=w519:errorcluster)  [unwired: 8 in]
                  n138 = call "MLLF_WriteToBuffer.vi"("String"=w517, "error in"=w519, "DriverConnect in"=w518) -> ("error out"=w524:T14, "DriverConnect out"=w523:T1)  [unwired: 5 in]
                  n139 = call "HDM3065B_ESR_check.vi"("Driver Name"=w521, "Error Code"=w522, "error in"=w524, "DriverConnect in"=w523) -> ("error out"=w520:T14)  [unwired: 6 in, 1 out]
                }
              }
            }
            frame #2 {
            }
          }
        }
        frame "get" {
          n140 = flat-sequence {
            tunnel: w544 -> [w554]
            tunnel: w545 -> [w555]
            tunnel: w546 -> [w556]
            tunnel: w535 -> [w549]
            tunnel: [w549] -> w543
            tunnel: [w556] -> w542
            tunnel: [w555] -> w541
            tunnel: [w553] -> w540
            tunnel: [w552] -> w539
            tunnel: [w550] -> w538
            tunnel: [w548] -> w537
            tunnel: [w554] -> w536
            tunnel: w534 -> [w551]
            tunnel: w543 -> [w567]
            tunnel: w542 -> [w565]
            tunnel: w541 -> [w564]
            tunnel: w540 -> [w562]
            tunnel: w539 -> [w561]
            tunnel: w538 -> [w560]
            tunnel: w537 -> [w559]
            tunnel: w536 -> [w557]
            tunnel: [w566] -> w533
            tunnel: [w563] -> w532
            tunnel: [w558] -> w531
            tunnel: [w600] -> w547
            tunnel: w533 -> [w600]
            tunnel: w532 -> [w598]
            tunnel: w531 -> [w599]
            tunnel: [w598] -> w530
            tunnel: [w599] -> w529
            frame #0 {
              n141 = Unbundle By Name(w549) -> ("Data.Connect"=w553:T1, "Data.Func"=w552:T7)
              n142 = call "MLLF_CommandDelimeter.vi"("command with param"=w551) -> ("command"=w550:string, "Spit delimetre"=w548:string)  [unwired: 6 in, 3 out]
            }
            frame #1 {
              n143 = case shown="\"TIMEOUT\"" w560 {
                selector: w560 -> [w570 _ _ _]
                tunnel: [w569 w574 w580 w587] -> w563
                tunnel: w565 -> [_ _ _ _]
                tunnel: [w571 w575 w586 w595] -> w566
                tunnel: w567 -> [w571 w575 w586 w595]
                tunnel: w562 -> [_ _ w579 w594]
                tunnel: w564 -> [_ _ _ _]
                tunnel: w559 -> [_ _ _ w589]
                tunnel: w561 -> [_ _ _ w593]
                tunnel: ["" ("String") w572 w576 w588] -> w558
                tunnel: w557 -> [_ w574 _ _]
                frame "False", Default {
                  n144 = call "MLLF_UnknownCommand(SubVI).vi"("Unknown command"=w570) -> ("error out"=w569:errorcluster)  [unwired: 10 in]
                }
                frame "TIMEOUT" {
                  n145 = Unbundle By Name(w575) -> ("Data.Connect.InterfaceSettings.TMO, ms"=w573:i32)
                  n146 = Format Value(value (0)=w573) -> (output string=w572:string)  [unwired: 2 in]
                }
                frame "READ" {
                  n147 = call "MLLF_WriteToBufferWithDelay.vi"("Delay Time ( 0,05 s)"=0.1 ("Delay Time (s)"), "Command"="READ?" ("String"), "DriverConnect in"=w579) -> ("Error Out"=w585:errorcluster, "DriverConnect out"=w584:T1)  [unwired: 7 in]
                  n148 = call "MLLF_ReadBuffer.vi"("Error In"=w585, "DriverConnect in"=w584) -> ("Error Out"=w580:errorcluster, "String"=w581:string)  [unwired: 6 in, 1 out]
                  n149 = Fract/Exp String To Number(use system decimal point (T)=FALSE, string=w581) -> (number=w577:dbl)  [unwired: 2 in, 1 out]
                  n150 = Format Value(value (0)=w577) -> (output string=w576:string)  [unwired: 2 in]
                }
                frame "SCPI" {
                  n151 = case shown="\"VDC\", Default" w593 {
                    tunnel: [1.0 ("Delay Time (s)") 0.05 ("Delay Time (s)")] -> w590
                    frame "F" {
                    }
                    frame "VDC", Default {
                    }
                  }
                  n152 = call "MLLF_WriteToBufferWithDelay.vi"("Delay Time ( 0,05 s)"=w590, "Command"=w589, "DriverConnect in"=w594) -> ("Error Out"=w592:errorcluster, "DriverConnect out"=w591:T1)  [unwired: 7 in]
                  n153 = call "MLLF_ReadBuffer.vi"("Error In"=w592, "DriverConnect in"=w591) -> ("Error Out"=w587:errorcluster, "String"=w588:string)  [unwired: 6 in, 1 out]
                }
              }
            }
            frame #2 {
            }
          }
        }
        frame "close" {
          n154 = Unbundle By Name(w602) -> ("Data.Connect.OpenedSession"=w604:T3)
          n155 = VISA Close(VISA resource name=w604) -> (error out=w603:errorcluster)  [unwired: 1 in]
        }
      }
    }
    frame Error {
    }
  }
  n156 = local write "Settings"(w1) -> ()
  n157 = flat-sequence {
    tunnel: [w616] -> w2
    tunnel: [w615] -> w4
    tunnel: w7 -> [w614]
    tunnel: w5 -> [w613]
    tunnel: w6 -> [w609]
    tunnel: [w611] -> w3
    frame #0 {
      # "driver out"
      n158 = Unbundle By Name(w609) -> ("Data"=w608:cluster{"Connect":T1, "Channel":T6, "Func":T7})
      n159 = To Variant(anything=w608) -> (Variant=w610:variant)
      n160 = Bundle By Name(cluster=w609, "Saved Data"=w610) -> (w611:T8)
      n161 = call "MLLF_SaveLastSettingUtility.vi"("error in"=w613, "Saved Data"=w610) -> ("error out"=w612:T14)  [unwired: 8 in, 1 out]
      n162 = call "MCF_Output.vi"("Error In"=w612, "Input"=w614) -> ("Error Out"=w615:errorcluster, "Output"=w616:string)  [unwired: 8 in]
    }
  }
  n163 = local write "Settings"(w3) -> ()
  "error out" <- w4
  "Response" <- w2
